vi "4.4_PH.vi"() -> ()   [LabVIEW 2023]
panel:
  out "pole powierzcni kuli":dbl
  out "objetosc kuli":dbl
  out "objetosc walca":dbl
  out "pole kola":dbl
  in  "wysokosc walca":dbl
  in  "promien podstawy - kola":dbl
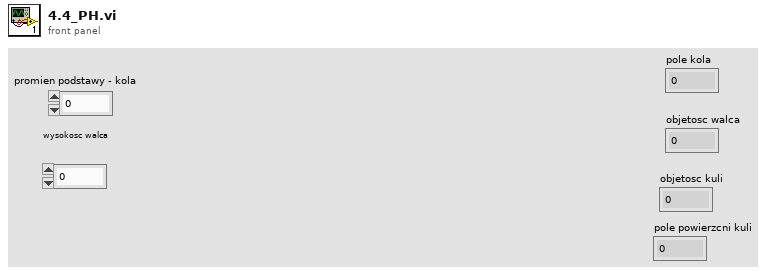
[diagram p1: front panel]
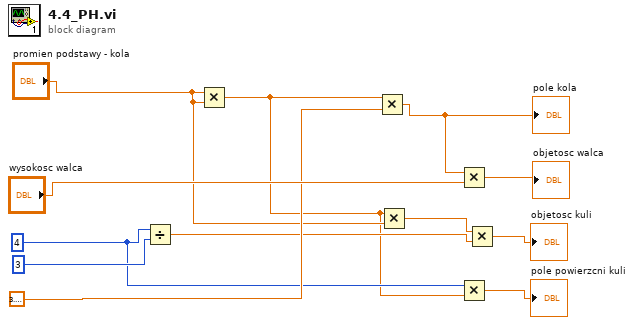
[diagram p0: block diagram]
diagram:
  w2 = 4
  n1 = Divide(x=w2, y=3) -> (x/y=w6:dbl)
  n2 = Multiply(x="promien podstawy - kola", y="promien podstawy - kola") -> (x*y=w1:dbl)
  n3 = Multiply(x=w1, y=3.141592653589793) -> (x*y=w12:dbl)
  "pole kola" <- w12
  n4 = Multiply(x=w1, y="promien podstawy - kola") -> (x*y=w5:dbl)
  n5 = Multiply(x=w12, y="wysokosc walca") -> (x*y=→"objetosc walca":dbl)
  n6 = Multiply(x=w2, y=w1) -> (x*y=→"pole powierzcni kuli":dbl)
  n7 = Multiply(x=w5, y=w6) -> (x*y=→"objetosc kuli":dbl)
